vi "NCS_AmpPh2.vi"(7 "Low-Pass Freq":dbl=200.0 format="%#_13g", 8 "IQ":cdb[](array[numeric]), 9 "data":cdb[][](array[numeric]), 10 "Sampling Rate":i32=500, 11 "Coerced Rx IQ Rate":dbl) -> (0 "Phase DownSampled":dbl[](array[numeric]), 1 "Amp DownSampled":dbl[](array[numeric]), 2 "Phase":dbl[](array[numeric]), 3 "Amplitude":dbl[](array[numeric]), 5 "Decimation Factor":dbl)   [LabVIEW 2016]
uses:
  <vilib>/Analysis/coordinate.llb/Wrap Angle (array).vi
  <vilib>/Analysis/3filter.llb/Butterworth Filter (DBL).vi
  <vilib>/Analysis/NI_AALBase.lvlib
  <vilib>/Analysis/NI_AALPro.lvlib
  <vilib>/Analysis/NI_AAL_Angle.lvlib
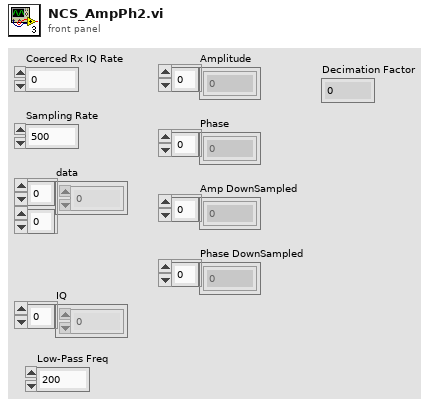
[diagram p1: front panel]
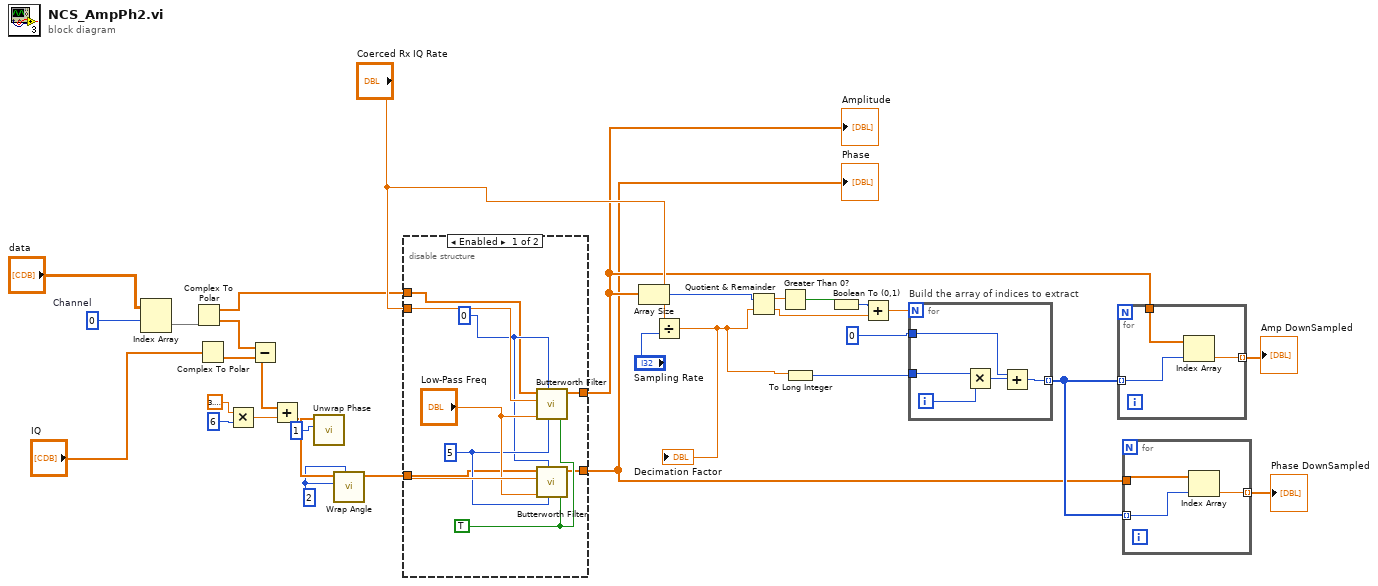
[diagram p0: block diagram]
diagram:
  w17 = 0  # Channel
  w28 = 2 ("y")
  n1 = Index Array(array="data", index (row)=w17) -> (element=w15:cdb[])  [unwired: 1 in]
  n2 = Complex To Polar(r * e^(i*theta)=w15) -> (r=w19:dbl[], theta=w30:dbl[])
  n3 = Complex To Polar(r * e^(i*theta)="IQ") -> (theta=w24:dbl[])  [unwired: 1 out]
  n4 = Multiply(x=3.141592653589793, y=6) -> (x*y=w23:dbl)
  n5 = Subtract(x=w30, y=w24) -> (x-y=w26:dbl[])
  n6 = Add(x=w26, y=w23) -> (x+y=w27:dbl[])
  n7 = call <vilib>:"Unwrap Phase.vi"("phase unit"=1 ("y"), "Phase"=w27) -> ("Unwrapped Phase"=w29:dbl[])  [unwired: 8 in, 1 out]
  n8 = call-poly <vilib>:"Wrap Angle.vi"("angle units"=w28, "angle range"=w28, "Angle In"=w29) -> ("Angle Out"=w31:dbl[])  [unwired: 7 in, 1 out]
  n9 = disable-structure shown="Enabled" {
    disable-tunnel: "Coerced Rx IQ Rate" -> [w41 _]
    disable-tunnel: w31 -> [w36 w42]
    disable-tunnel: w19 -> [w35 w43]
    disable-tunnel: [w34 w43] -> w5
    disable-tunnel: [w33 w42] -> w2
    frame Enabled {
      w38 = 5 ("order1")
      w39 = TRUE
      w37 = 0
      n10 = call-poly <vilib>:"Butterworth Filter.vi"("init/cont (init:F)"=w39, "order"=w38, "filter type"=w37, "low cutoff freq: fl"="Low-Pass Freq", "sampling freq: fs"=w41, "X"=w35) -> ("Filtered X"=w34:dbl[])  [unwired: 2 in, 1 out]
      n11 = call-poly <vilib>:"Butterworth Filter.vi"("init/cont (init:F)"=w39, "order"=w38, "filter type"=w37, "low cutoff freq: fl"="Low-Pass Freq", "sampling freq: fs"=w41, "X"=w36) -> ("Filtered X"=w33:dbl[])  [unwired: 2 in, 1 out]
    }
    frame Disabled {
    }
  }
  "Phase" <- w2
  "Amplitude" <- w5
  n12 = Array Size(array=w5) -> (size(s)=w14:i32)
  n13 = Divide(x="Coerced Rx IQ Rate", y="Sampling Rate") -> (x/y=w7:dbl)
  "Decimation Factor" <- w7
  n14 = Quotient & Remainder(x=w14, y=w7) -> (x-y*floor(x/y)=w13:dbl, floor(x/y)=w9:dbl)
  n15 = Greater Than 0?(x=w13) -> (x > 0?=w10:bool)
  n16 = To Long Integer(number=w7) -> (32bit integer=w6:i32)
  n17 = Boolean To (0,1)(Boolean=w10) -> (0, 1=w12:i16)
  n18 = Add(x=w12, y=w9) -> (x+y=w11:dbl)
  n19 = for "Build the array of indices to extract" {
    N: w11 -> [_]
    tunnel: w6 -> [w45]
    tunnel: 0 -> [w48]
    tunnel: [w44] -> w3 mode=indexing
    i -> [w47]
    n20 = Multiply(x=w45, y=w47) -> (x*y=w46:i32)
    n21 = Add(x=w48, y=w46) -> (x+y=w44:i32)
  }
  n22 = for {
    tunnel: w3 -> [w50] mode=indexing
    tunnel: w5 -> [w51]
    tunnel: [w49] -> w4 mode=indexing
    n23 = Index Array(array=w51, index=w50) -> (element=w49:dbl)
  }
  "Amp DownSampled" <- w4
  n24 = for {
    tunnel: w3 -> [w53] mode=indexing
    tunnel: w2 -> [w54]
    tunnel: [w52] -> w1 mode=indexing
    n25 = Index Array(array=w54, index=w53) -> (element=w52:dbl)
  }
  "Phase DownSampled" <- w1
